vi "Get_MPUTemp.vi"(5 "Device Number":T1, 7 "Update":bool) -> (2 "MPUTemp":dbl)   [LabVIEW 2019]
doc: "This navX VI returns the current MPU Temperature."
uses:
  <vilib>/Rock Robotics/WPI/ThirdParty/Sensors/navX/_TypeDefs/FRIC_navX_DeviceNumbersTypeDef.ctl
  <vilib>/Rock Robotics/WPI/ThirdParty/Sensors/navX/_TypeDefs/Z900_navX_DeviceRegisters.ctl
  <vilib>/Rock Robotics/WPI/ThirdParty/Sensors/navX/_Util/Z900_navX_Util_LittleEndian_to_BigEndian.vi
  <vilib>/Rock Robotics/WPI/ThirdParty/Sensors/navX/Get/_Internal/FRIC_navX_Get_Registry.vi
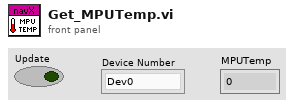
[diagram p1: front panel]
types:
  T1 = typedef "FRIC_navX_DeviceNumbersTypeDef.ctl" = enum16{"Dev0", "Dev1", "Dev2", "Dev3"}
  T2 = typedef "Z900_navX_DeviceRegisters.ctl" = u8
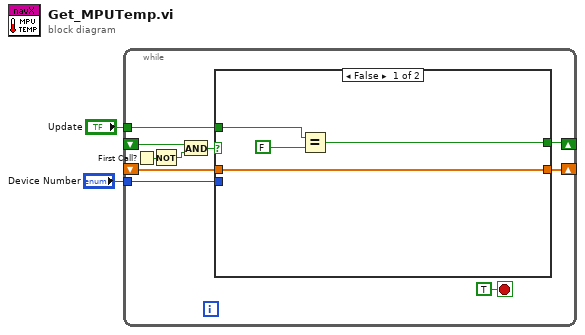
[diagram p0: block diagram]
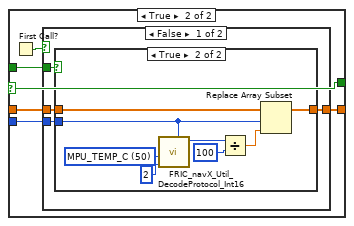
[diagram p2: hidden frame]
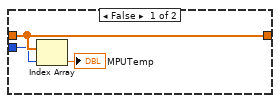
[diagram p3: hidden frame]
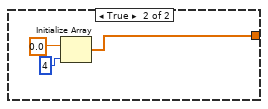
[diagram p4: hidden frame]
diagram:
  n1 = while {
    shift-right: [w12] -> _
    shift-left: _ -> [w9]
    tunnel: "Update" -> [w10]
    tunnel: "Device Number" -> [w8]
    shift-right: [w3] -> _
    shift-left: _ -> [w5]
    stop <- TRUE stop-if-true
    n2 = First Call?() -> (First Call?: T/F=w6:bool)
    n3 = Not(x=w6) -> (.not. x?=w7:bool)
    n4 = And(x=w5, y=w7) -> (x .and. y?=w4:bool)
    n5 = case shown="False" w4 {
      selector: w4 -> [_ w17]
      tunnel: [w16 w22] -> w12
      tunnel: w10 -> [w14 w21]
      tunnel: w9 -> [w16 w20]
      tunnel: w8 -> [_ w19]
      tunnel: [w13 w17] -> w3
      frame False {
        n6 = Equal?(x=w14, y=FALSE) -> (x = y?=w13:bool)
      }
      frame True {
        n7 = First Call?() -> (First Call?: T/F=w18:bool)
        n8 = case shown="False" w18 {
          tunnel: [w26 w40] -> w22
          tunnel: w21 -> [w25 _]
          tunnel: w20 -> [w24 _]
          tunnel: w19 -> [w23 _]
          frame False {
            n9 = case shown="True" w25 {
              tunnel: [w28 w32] -> w26
              tunnel: w24 -> [w28 w33]
              tunnel: w23 -> [w27 w30]
              frame False {
                n10 = Index Array(array=w28, index=w27) -> (element=→"MPUTemp":dbl)
              }
              frame True {
                w35 = T2 50 items=["WHOAMI"=0, "HW_REV"=1, "FW_VER_MAJOR"=2, "FW_VER_MINOR"=3, "UPDATE_RATE_HZ"=4, "ACCEL_FSR_G"=5, "GYRO_FSR_DPS"=6, "OP_STATUS"=8, "CAL_STATUS"=9, "SELFTEST_STATUS"=10, "CAPABILITY_FLAGS_L"=11, "CAPABILITY_FLAGS_H"=12, "SENSOR_STATUS"=16, "TIMESTAMP"=18, "YAW"=22, "ROLL"=24, "PITCH"=26, "HEADING"=28, "FUSED_HEADING"=30, "ALTITUDE_I"=32, "ALTITUDE_D"=34, "LINERA_ACC_X"=36, "LINERA_ACC_Y"=38, "LINERA_ACC_Z"=40, "QUAT_W"=42, "QUAT_X"=44, "QUAT_Y"=46, "QUAT_Z"=48, "MPU_TEMP_C"=50, "GYRO_X"=52, "GYRO_Y"=54, "GYRO_Z"=56, "ACC_X"=58, "ACC_Y"=60, "ACC_Z"=62, "MAG_X"=64, "MAG_Y"=66, "MAG_Z"=68, "PRESSURE_I"=70, "PRESSURE_D"=72, "PRESSURE_TEMP"=74, "YAW_OFFSET"=76, "QUAT_OFFSET_W"=78, "QUAT_OFFSET_X"=80, "QUAT_OFFSET_Y"=82, "QUAT_OFFSET_Z"=84, "INTEGRATION_CONTROL"=86, "VELOCITY_X"=88, "VELOCITY_Y"=92, "VELOCITY_Z"=96, "DISPLACMENT_X"=100, "DISPLACMENT_Y"=104, "DISPLACEMENT_Z"=108] ("Device Register")
                n11 = call <vilib>:"FRIC_navX_Util_DecodeProtocol_Int16.vi"("Device Number"=w30, "length"=2, "Device Register"=w35) -> ("Value"=w36:i16)  [unwired: 8 in]
                n12 = Divide(x=w36, y=100) -> (x/y=w31:dbl)
                n13 = Replace Array Subset(array=w33, new element=w31, index=w30) -> (w32:dbl[])
              }
            }
          }
          frame True {
            n14 = Initialize Array(0.0, 4 ("dimension size")) -> (w40:dbl[])
          }
        }
      }
    }
  }
